vi "Initialize.vi"(8 "error in":errorcluster, 11 "Plugin in":refnum<class "PXIe4113 DUT Power Control Replacement.lvclass">) -> (0 "error out":errorcluster, 3 "Plugin out":refnum<class "PXIe4113 DUT Power Control Replacement.lvclass">)   [LabVIEW 2026, in "PXIe4113 DUT Power Control Replacement.lvlib" / "PXIe4113 DUT Power Control Replacement.lvclass"]
uses:
  PXIe4113 DUT Power Control Replacement.lvclass
  C:/Program Files/National Instruments/LabVIEW 2026/vi.lib/FlexLogger/SDK/PluginSDK.lvlibp/PEFClasses/SDK/Plugin/Plugin.lvclass
  <vilib>/FlexLogger/SDK/PluginSDK.lvlibp/PEFClasses/SDK/Setpoint Consumer Channel/Setpoint Consumer Channel.lvclass
  C:/Program Files/National Instruments/LabVIEW 2026/vi.lib/FlexLogger/SDK/PluginSDK.lvlibp/PEFClasses/SDK/Channel/Channel.lvclass
  <vilib>/FlexLogger/SDK/PluginSDK.lvlibp/PEFClasses/SDK/Producer Channel/Producer Channel.lvclass
  <vilib>/FlexLogger/SDK/PluginSDK.lvlibp/PEFClasses/SDK/Plugin/ParameterAccess/Write String.vi
  <vilib>/FlexLogger/SDK/PluginSDK.lvlibp/PEFClasses/SDK/Setpoint Consumer Channel/Create Setpoint Consumer Channel.vi
  <vilib>/FlexLogger/SDK/PluginSDK.lvlibp/PEFClasses/SDK/Producer Channel/Create Producer Channel_v2.vi
  <vilib>/FlexLogger/SDK/PluginSDK.lvlibp/PEFClasses/SDK/Plugin/Plugin.lvclass
  C:/Program Files/National Instruments/LabVIEW 2026/vi.lib/FlexLogger/SDK/PluginSDK.lvlibp/PEFClasses/SDK/Processing Element/Processing Element.lvclass
  C:/Users/localadmin/Documents/LabVIEW Projects/FlexLogger IO Plug-ins/PXIe4113 DUT Power Control Replacement/PXIe4113 DUT Power Control Replacement.lvclass
  <vilib>/FlexLogger/SDK/PluginSDK.lvlibp
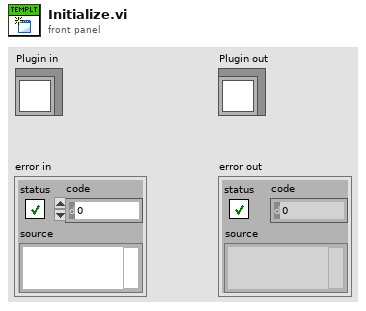
[diagram p1: front panel]
types:
  T1 = cluster{"Timing Method":enum16{"Periodic", "Immediate", "On Data Ready", "Triggered"}, "Timing Period (ms)":i32}
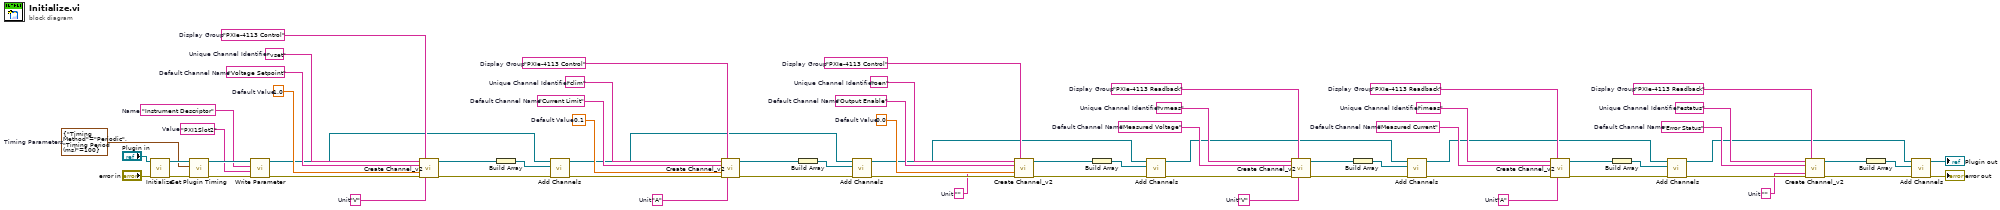
[diagram p0: block diagram]
diagram:
  w7 = ""  # Unit
  w8 = "PXIe-4113 Readback"  # Display Group
  w10 = "Error Status"  # Default Channel Name
  w11 = "estatus"  # Unique Channel Identifier
  w16 = "A"  # Unit
  w17 = "PXIe-4113 Readback"  # Display Group
  w19 = "Measured Current"  # Default Channel Name
  w20 = "imeas"  # Unique Channel Identifier
  w25 = "V"  # Unit
  w26 = "PXIe-4113 Readback"  # Display Group
  w28 = "Measured Voltage"  # Default Channel Name
  w29 = "vmeas"  # Unique Channel Identifier
  w37 = 0.0  # Default Value
  w34 = ""  # Unit
  w35 = "PXIe-4113 Control"  # Display Group
  w38 = "Output Enable"  # Default Channel Name
  w39 = "oen"  # Unique Channel Identifier
  w47 = 0.1  # Default Value
  w44 = "A"  # Unit
  w45 = "PXIe-4113 Control"  # Display Group
  w48 = "Current Limit"  # Default Channel Name
  w49 = "clim"  # Unique Channel Identifier
  w57 = 1.0  # Default Value
  w54 = "V"  # Unit
  w55 = "PXIe-4113 Control"  # Display Group
  w58 = "Voltage Setpoint"  # Default Channel Name
  w59 = "vset"  # Unique Channel Identifier
  w61 = "PXI1Slot2"  # Value
  w62 = "Instrument Descriptor"  # Name
  w65 = T1 {"Timing Method"=enum."Periodic", "Timing Period (ms)"=100}  # Timing Parameters
  n1 = call-parent "Initialize.vi"("error in (no error)"="error in", "Plugin in"="Plugin in") -> ("error out"=w64:errorcluster, "Plugin out"=w66:refnum<class "PXIe4113 DUT Power Control Replacement.lvclass">)  [unwired: 8 in]
  n2 = call <vilib>:"Set Plugin Timing.vi"("error in (no error)"=w64, "Timing Parameters"=w65, "Plugin in"=w66) -> ("error out"=w60:errorcluster, "Plugin out"=w63:refnum<class "PXIe4113 DUT Power Control Replacement.lvclass">)  [unwired: 7 in]
  n3 = call-poly <vilib>:"Write Parameter.vi"("error in (no error)"=w60, "Value"=w61, "Name"=w62, "Plugin in"=w63) -> ("error out"=w56:errorcluster, "Plugin out"=w52:refnum<class "PXIe4113 DUT Power Control Replacement.lvclass">)  [unwired: 6 in]
  n4 = call-poly <vilib>:"Create Channel_v2.vi"("Unique Channel Identifier"=w59, "Display Group"=w55, "Default Channel Name"=w58, "Default Value"=w57, "error in (no error)"=w56, "Unit"=w54) -> ("Setpoint Consumer Channel"=w53:refnum<class "Setpoint Consumer Channel.lvclass">, "error out"=w50:errorcluster)  [unwired: 8 in]
  n5 = Build Array(w53) -> (w51:refnum<class "Setpoint Consumer Channel.lvclass">[])
  n6 = call <vilib>:"Add Channels.vi"("error in (no error)"=w50, "Channels"=w51, "Plugin in"=w52) -> ("error out"=w46:errorcluster, "Plugin out"=w42:refnum<class "PXIe4113 DUT Power Control Replacement.lvclass">)  [unwired: 7 in]
  n7 = call-poly <vilib>:"Create Channel_v2.vi"("Unique Channel Identifier"=w49, "Display Group"=w45, "Default Channel Name"=w48, "Default Value"=w47, "error in (no error)"=w46, "Unit"=w44) -> ("Setpoint Consumer Channel"=w43:refnum<class "Setpoint Consumer Channel.lvclass">, "error out"=w40:errorcluster)  [unwired: 8 in]
  n8 = Build Array(w43) -> (w41:refnum<class "Setpoint Consumer Channel.lvclass">[])
  n9 = call <vilib>:"Add Channels.vi"("error in (no error)"=w40, "Channels"=w41, "Plugin in"=w42) -> ("error out"=w36:errorcluster, "Plugin out"=w32:refnum<class "PXIe4113 DUT Power Control Replacement.lvclass">)  [unwired: 7 in]
  n10 = call-poly <vilib>:"Create Channel_v2.vi"("Unique Channel Identifier"=w39, "Display Group"=w35, "Default Channel Name"=w38, "Default Value"=w37, "error in (no error)"=w36, "Unit"=w34) -> ("Setpoint Consumer Channel"=w33:refnum<class "Setpoint Consumer Channel.lvclass">, "error out"=w30:errorcluster)  [unwired: 8 in]
  n11 = Build Array(w33) -> (w31:refnum<class "Setpoint Consumer Channel.lvclass">[])
  n12 = call <vilib>:"Add Channels.vi"("error in (no error)"=w30, "Channels"=w31, "Plugin in"=w32) -> ("error out"=w27:errorcluster, "Plugin out"=w23:refnum<class "PXIe4113 DUT Power Control Replacement.lvclass">)  [unwired: 7 in]
  n13 = call-poly <vilib>:"Create Channel_v2.vi"("Unique Channel Identifier"=w29, "Display Group"=w26, "Default Channel Name"=w28, "error in (no error)"=w27, "Unit"=w25) -> ("Producer Channel"=w24:refnum<class "Producer Channel.lvclass">, "error out"=w21:errorcluster)  [unwired: 9 in]
  n14 = Build Array(w24) -> (w22:refnum<class "Producer Channel.lvclass">[])
  n15 = call <vilib>:"Add Channels.vi"("error in (no error)"=w21, "Channels"=w22, "Plugin in"=w23) -> ("error out"=w18:errorcluster, "Plugin out"=w14:refnum<class "PXIe4113 DUT Power Control Replacement.lvclass">)  [unwired: 7 in]
  n16 = call-poly <vilib>:"Create Channel_v2.vi"("Unique Channel Identifier"=w20, "Display Group"=w17, "Default Channel Name"=w19, "error in (no error)"=w18, "Unit"=w16) -> ("Producer Channel"=w15:refnum<class "Producer Channel.lvclass">, "error out"=w12:errorcluster)  [unwired: 9 in]
  n17 = Build Array(w15) -> (w13:refnum<class "Producer Channel.lvclass">[])
  n18 = call <vilib>:"Add Channels.vi"("error in (no error)"=w12, "Channels"=w13, "Plugin in"=w14) -> ("error out"=w9:errorcluster, "Plugin out"=w5:refnum<class "PXIe4113 DUT Power Control Replacement.lvclass">)  [unwired: 7 in]
  n19 = call-poly <vilib>:"Create Channel_v2.vi"("Unique Channel Identifier"=w11, "Display Group"=w8, "Default Channel Name"=w10, "error in (no error)"=w9, "Unit"=w7) -> ("Producer Channel"=w6:refnum<class "Producer Channel.lvclass">, "error out"=w3:errorcluster)  [unwired: 9 in]
  n20 = Build Array(w6) -> (w4:refnum<class "Producer Channel.lvclass">[])
  n21 = call <vilib>:"Add Channels.vi"("error in (no error)"=w3, "Channels"=w4, "Plugin in"=w5) -> ("error out"=→"error out":errorcluster, "Plugin out"=→"Plugin out":refnum<class "PXIe4113 DUT Power Control Replacement.lvclass">)  [unwired: 7 in]
